vi "PulsePlusOne.vi"(2 "error in":errorcluster, 3 "Tree Name":string="proto_tree") -> (0 "error out":errorcluster, 1 "Shot #":i32)   [LabVIEW 2011]
uses:
  <vilib>/MDSplus/Library/MDSplus.lvlib
  <vilib>/MDSplus/Classes/Tree_Class/Tree.lvclass
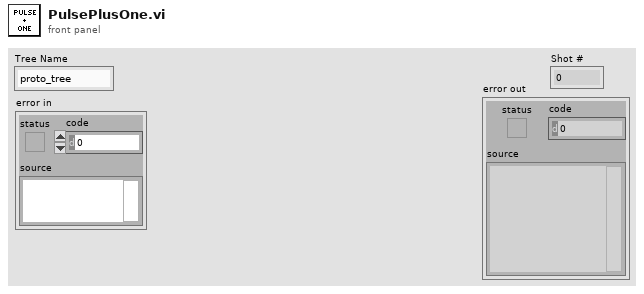
[diagram p1: front panel]
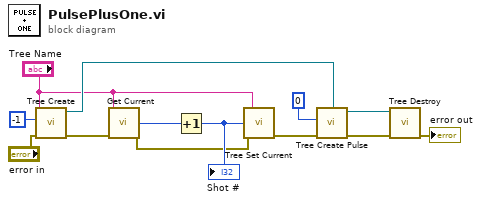
[diagram p0: block diagram]
diagram:
  n1 = call <vilib>:"Tree Create.vi"("error in (no error)"="error in", "Shot"=-1, "Name"="Tree Name") -> ("error out"=w10:errorcluster, "Tree DVR out"=w4:refnum<data-value>)  [unwired: 7 in]
  n2 = call <vilib>:"Get Current.vi"("error in (no error)"=w10, "Tree name"="Tree Name") -> ("error out"=w7:errorcluster, "Current shot out"=w9:i32)  [unwired: 7 in, 1 out]
  n3 = Increment(x=w9) -> (x+1=w8:i32)
  "Shot #" <- w8
  n4 = call <vilib>:"Tree Set Current.vi"("error in (no error)"=w7, "Shot"=w8, "Tree name"="Tree Name") -> ("error out"=w5:errorcluster)  [unwired: 7 in, 1 out]
  n5 = call <vilib>:"Tree Create Pulse.vi"("error in (no error)"=w5, "Shot"=0, "Tree DVR in"=w4) -> ("error out"=w12:errorcluster, "Tree DVR out"=w11:refnum<data-value>)  [unwired: 7 in]
  n6 = call <vilib>:"Tree Destroy.vi"("error in (no error)"=w12, "Tree DVR in"=w11) -> ("error out"=→"error out":errorcluster)  [unwired: 9 in]
